vi "_Get or Add SharedStringTablePart.vi"(8 "error in":errorcluster, 11 "SpreadsheetDoument in":refnum<k24>) -> (0 "error out":errorcluster, 2 "SharedStringTablePart":refnum<k24>, 3 "SpreadsheetDocument out":refnum<k24>)   [LabVIEW 2021, in "Open Xml.lvlib"]
uses:
  Open Xml.lvlib
  D:/git/Open-Xml-LabVIEW/dll/DocumentFormat.OpenXml.dll
  dll/DocumentFormat.OpenXml.dll
  D:/git/Open-Xml-LabVIEW/dll/OpenXmlGenericsWrapper.dll
  dll/OpenXmlGenericsWrapper.dll
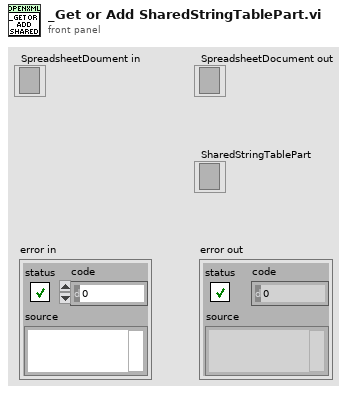
[diagram p1: front panel]
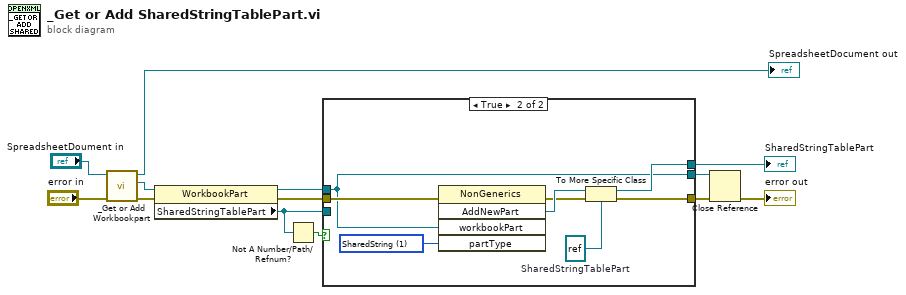
[diagram p0: block diagram]
diagram:
  n1 = call "_Get or Add Workbookpart.vi"("error in"="error in", "SpreadsheetDocument"="SpreadsheetDoument in") -> ("error out"=w7:errorcluster, "WorkbookPart"=w3:refnum<k24>, "SpreadsheetDocument out"=→"SpreadsheetDocument out":refnum<k24>)  [unwired: 7 in]
  n2 = property class="WorkbookPart"(reference=w3, error in=w7) -> (reference out=w4:refnum<k24>, error out=w11:errorcluster, "SharedStringTablePart"=w10:refnum<k24>)
  n3 = Not A Number/Path/Refnum?(number/path/refnum=w10) -> (NaN/Path/Refnum?=w12:bool)
  n4 = case shown="True" w12 {
    tunnel: w4 -> [w14 w17]
    tunnel: w11 -> [w15 w24]
    tunnel: w10 -> [w16 _]
    tunnel: [w16 w21] -> w8
    tunnel: [w15 w20] -> w9
    tunnel: [w14 w17] -> w1
    frame False {
    }
    frame True {
      w19 = refnum<k24> refnum  # SharedStringTablePart
      w23 = 1 items=["Worksheet", "SharedString"] ("partType")
      # "workbookPart.AddNewPart<SharedStringTablePart>();"
      n5 = invoke class="NonGenerics" method="AddNewPart"(error in=w24, "workbookPart"=w17, "partType"=w23) -> (error out=w18:errorcluster, "AddNewPart"=w22:refnum<k24>)  [unwired: 2 in, 3 out]
      n6 = To More Specific Class(target class=w19, reference=w22, error in=w18) -> (specific class reference=w21:refnum<k24>, error out=w20:errorcluster)
    }
  }
  "SharedStringTablePart" <- w8
  n7 = Close Reference(reference=w1, error in (no error)=w9) -> (error out=→"error out":errorcluster)
